vi "movimentacao_cin_inv.vi"() -> ()   [LabVIEW 2017]
doc: "The myRIO Project template acquires acceleration data from the onboard accelerometer and displays the changes of acceleration values in a waveform chart."
uses:
  <vilib>/myRIO/Instrument Drivers/Onboard IO/PWM/PWM.lvlib
  <vilib>/myRIO/Instrument Drivers/Onboard IO/PWM/typedefs/PWM Configuration.ctl
  <vilib>/myRIO/Common/Instrument Driver Framework/myRIO v1.0/PWM/typedefs/PWM Channels Enum.ctl
  <vilib>/myRIO/Common/Instrument Driver Framework/Utilities/typedefs/Generic FPGA Reference.ctl
  <vilib>/myRIO/Common/Instrument Driver Framework/Utilities/typedefs/myRIO v1.0 Reference.ctl
  <vilib>/myRIO/Common/Instrument Driver Framework/Utilities/typedefs/Hardware Version Enum.ctl
  <vilib>/myRIO/Common/Instrument Driver Framework/Utilities/typedefs/myRIO Generic Hardware Reference.ctl
  <vilib>/myRIO/Instrument Drivers/Onboard IO/PWM/typedefs/PWM Reference.ctl
  <vilib>/userdefined/High Color/nirio_resource_hc.ctl
  <vilib>/myRIO/Common/Instrument Driver Framework/myRIO v1.0/PWM/vis/myRIO v1.1 Open PWM.vi
  <vilib>/myRIO/Instrument Drivers/Onboard IO/PWM/vis/myRIO PWM Open.xnode
  <vilib>/Analysis/Matrix/Datatypes/RealMatrix.ctl
  <vilib>/Analysis/Matrix/NI_Matrix.lvlib
panel:
  in  "número de pontos que a matriz deve retornar":i64
  in  "String 2":string="(151,57;2,89;11,57);(245,79;-185,54;30);(126,28;-267,6;41,68);(43,16; -253,15;220,9);(-167,79;-132,49;100)"
  out "output array":T1
  out "appended array 2":dbl[](array[numeric])
  out "logical AND":bool
  out "x = y?":bool[](array[boolean])
  out "POS_E_ORIEN_HOME":dbl[](array[numeric])
  out "ANG_POSI_E_ORIEN_HOME":dbl[](array[numeric])
  out "CURRENT POSITIONS OF THE MOTORS":dbl[](array[numeric])
  in  "angulo_garra":dbl(knob) scale=-180.0..180.0
  out "POSITIONS SEQUENCE":T1
  in  "Duty Cycle Abert":dbl=0.04 format="%#_13g"
  out "Actuator 2":bool
  in  "Actuator":bool
  in  "Conveyor speed (mm/s)":dbl(slide)=200.0 step=1.0 scale=0.0..350.0
  out "indexador":i32
  out "Objeto detectado":bool
  out "Manipulando":bool
  out "Está em Home":bool
  out "Posicao_desejada":bool
  in  "Home":bool
  in  "error in (no error)":errorcluster
  in  "PARAR":bool
  in  "POSITION VECTOR":dbl[](array[numeric])
  # "ROTINA DE CONTROLE DO PROTÓTIPO DE FMS"
  # "COMANDO DE POSIÇÃO\nATUAL DOS MOTORES"
  # "OPERATION STATUS"
  # "ÂNGULOS DE JUNTAS"
  # "THETA 1"
  # "MOTOR 1"
  # "HOME"
  # "THETA 2"
  # "MOTOR 2"
  # "DESIRED POSITION"
  # "THETA 3"
  # "MOTOR 3"
  # "OBJECT DETECTED"
  # "THETA 4"
  # "MOTOR 4"
  # "MANIPULATING"
  # "THETA 5"
  # "MOTOR 5"
  # "ACTUATOR"
  # "MOTOR 6"
  # "VELOCIDADE DA ESTEIRA (mm/s)"
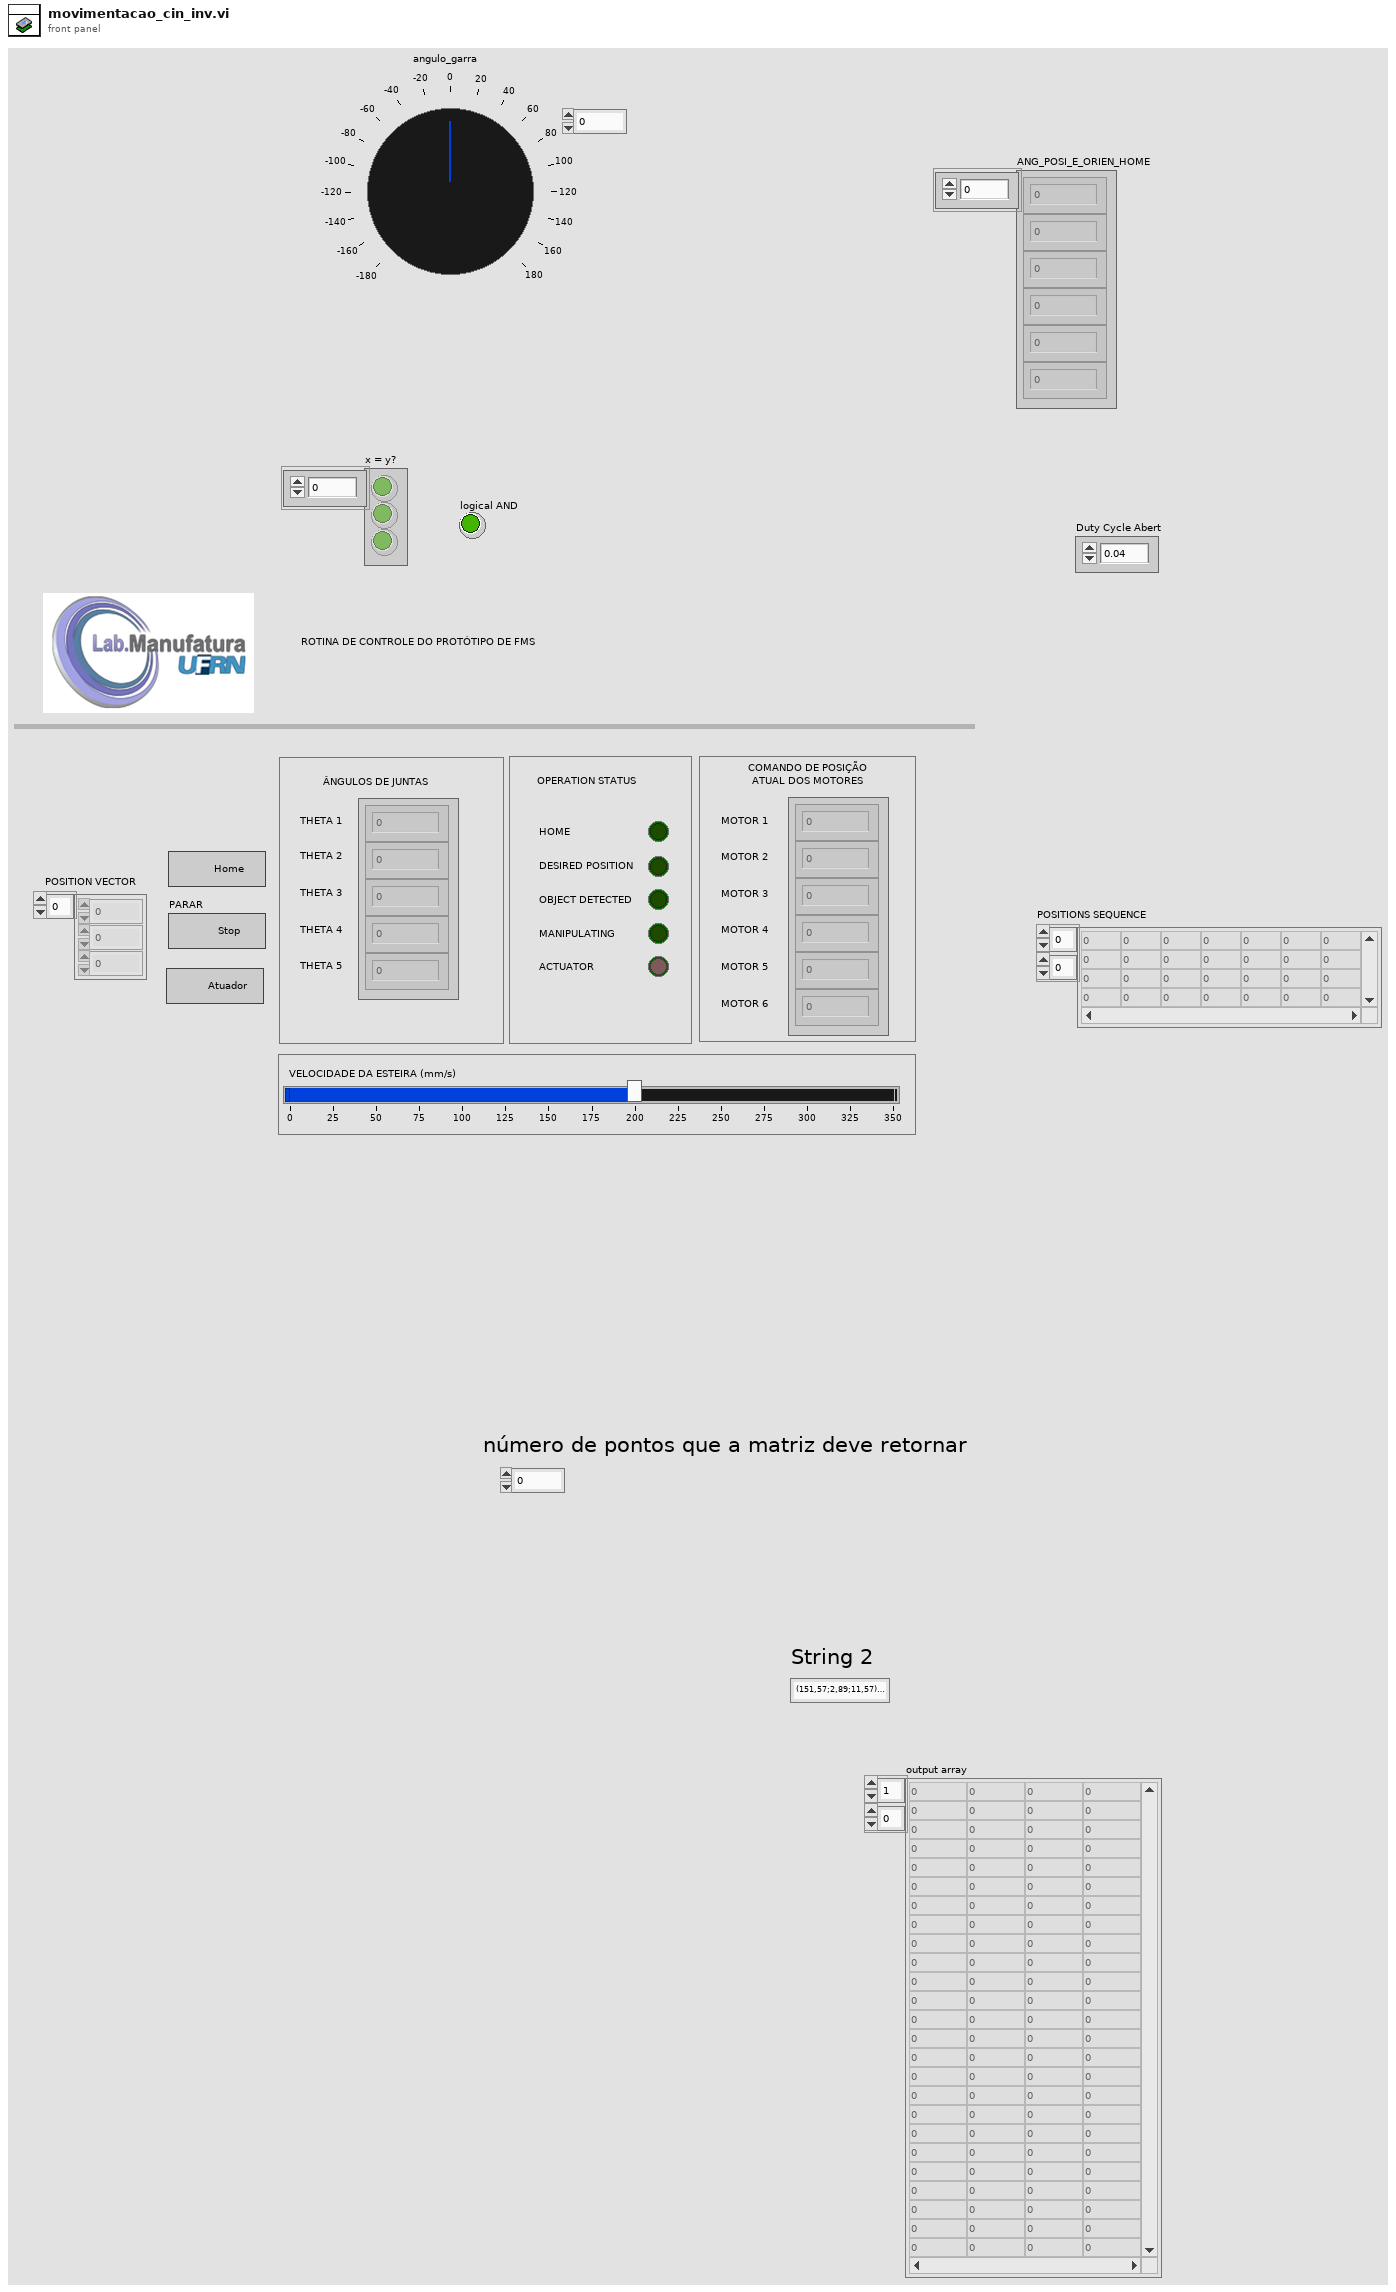
[diagram p1: front panel]
types:
  T1 = typedef "NI_Matrix.lvlib/RealMatrix.ctl" = dbl[][]
  T2 = cluster{"theta 1":dbl, "theta 2":dbl, "theta 3":dbl, "theta5":dbl, "theta4":dbl}
  T3 = typedef "nirio_resource_hc.ctl" = tag
  T4 = typedef "Hardware Version Enum.ctl" = enum16{"Unknown", "myRIO-1900", "myRIO-1950", "roboRIO", "NI ELVIS RIO CM"}
  T5 = typedef "PWM.lvlib/PWM Reference.ctl" = cluster{"myRIO Reference":T6, "PWM Channels Enum":T9, "PWM Configuration":T10}
  T6 = typedef "myRIO Generic Hardware Reference.ctl" = cluster{"myRIO Model":T4, "myRIO Hardware Reference":T7}
  T7 = typedef "myRIO v1.0 Reference.ctl" = cluster{"Generic FPGA Reference":T8, "Allow multiple opens":bool}
  T8 = typedef "Generic FPGA Reference.ctl" = refnum<k20>
  T9 = typedef "PWM Channels Enum.ctl" = enum16{"Not Connected", "C/PWM0", "C/PWM1", "A/PWM0", "A/PWM1", "A/PWM2", "B/PWM0", "B/PWM1", "B/PWM2", "PWM/PWM0", "PWM/PWM1", "PWM/PWM2", "PWM/PWM3", "PWM/PWM4", "PWM/PWM5", "PWM/PWM6", "PWM/PWM7", "PWM/PWM8", "PWM/PWM9"}
  T10 = typedef "PWM.lvlib/PWM Configuration.ctl" = cluster{"Frequency":dbl, "Duty Cycle":dbl}
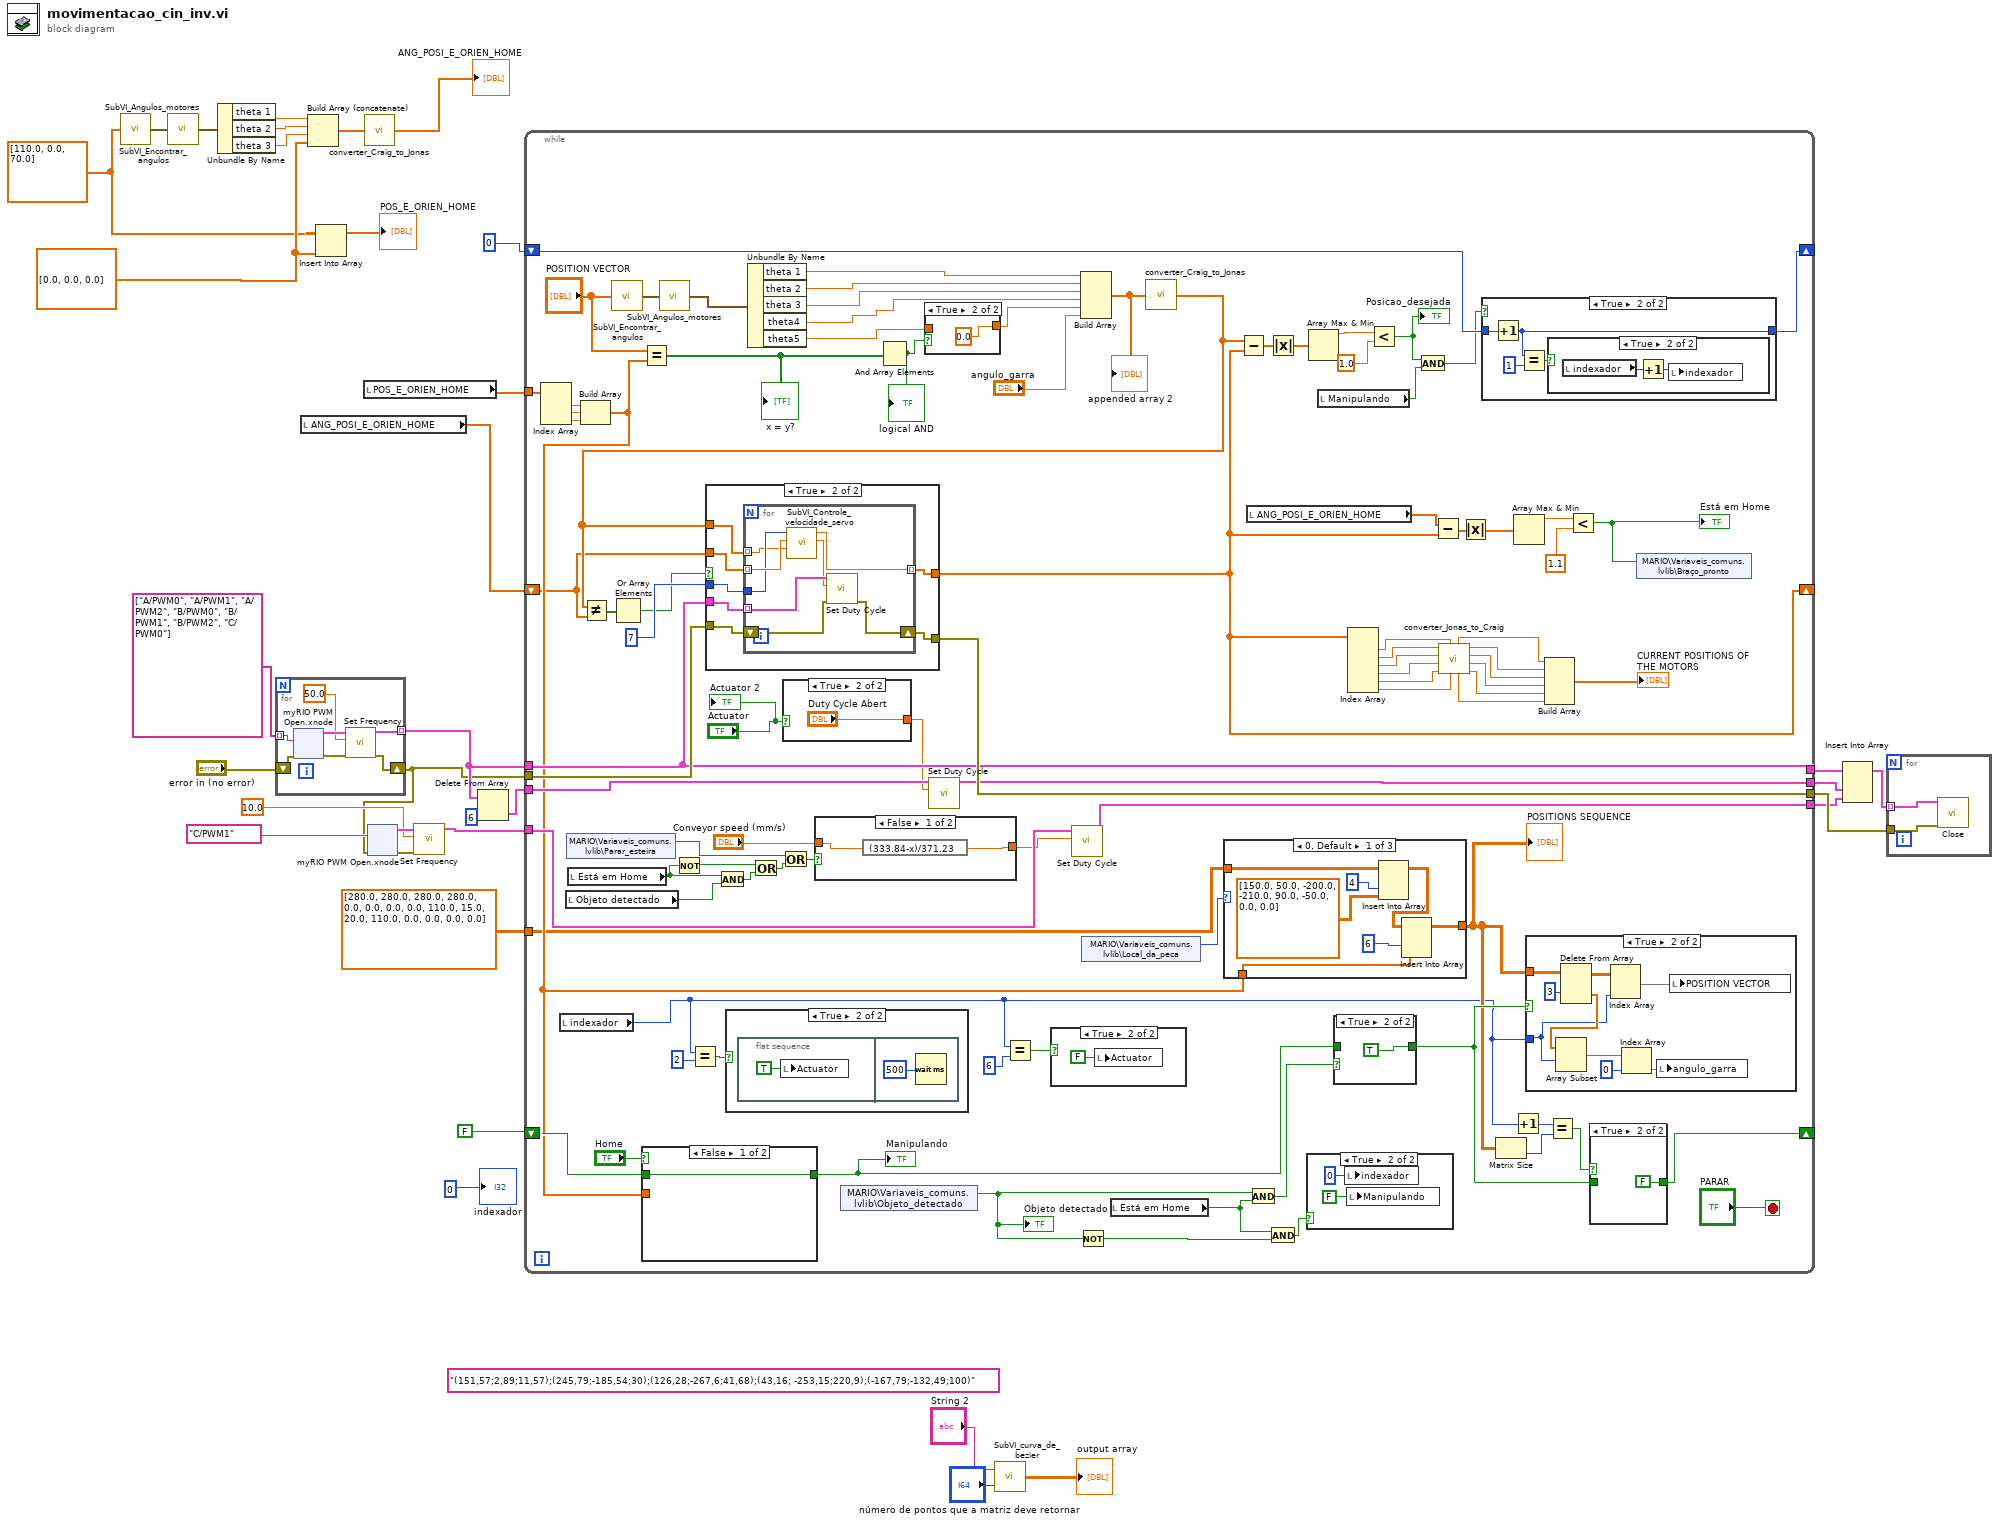
[diagram p0: block diagram]
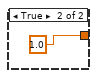
[diagram p2: hidden frame]
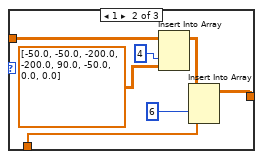
[diagram p4: hidden frame]
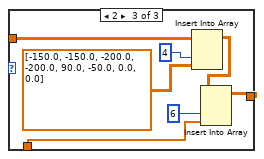
[diagram p5: hidden frame]
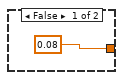
[diagram p7: hidden frame]
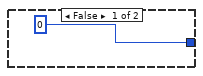
[diagram p11: hidden frame]
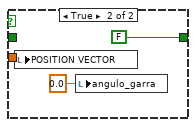
[diagram p15: hidden frame]
diagram:
  (unwired) "(151,57;2,89;11,57);(245,79;-185,54;30);(126,28;-267,6;41,68);(43,16; -253,15;220,9);(-167,79;-132,49;100)" ("String 2")
  w12 = dbl[] [0.0, 0.0, 0.0] ("vetor_P")
  w6 = dbl[] [110.0, 0.0, 70.0] ("vetor_P")
  n1 = call "SubVI_Encontrar_angulos.vi"("vetor_P"=w6) -> ("ângulos de Juntas"=w5:T2)
  n2 = call "SubVI_Angulos_motores.vi"("input cluster"=w5) -> ("output cluster"=w4:T2)
  n3 = Unbundle By Name(w4) -> ("theta 1"=w16:dbl, "theta 2"=w15:dbl, "theta 3"=w14:dbl)
  n4 = for {
    tunnel: tag[] ["A/PWM0", "A/PWM1", "A/PWM2", "B/PWM0", "B/PWM1", "B/PWM2", "C/PWM0"] -> [w39] mode=indexing
    tunnel: [w38] -> w29 mode=indexing
    shift-right: [w37] -> w18
    shift-left: "error in (no error)" -> [w36]
    n5 = xnode ("myRIO PWM Open.xnode")("error in (no error)"=w36, "Channel Name"=w39) -> ("error out"=w40:errorcluster, "PWM Ref Out"=w42:T5)  [unwired: 1 in]
    n6 = call <vilib>:"Set Frequency.vi"("error in (no error)"=w40, "Frequency [Hz]"=50.0, "PWM Ref In"=w42) -> ("error out"=w37:errorcluster, "PWM Ref Out"=w38:T5)  [unwired: 6 in]
  }
  n7 = local read "ANG_POSI_E_ORIEN_HOME"() -> (w13:dbl[])
  n8 = Build Array (concatenate)(w16, w15, w14, w12) -> (w8:dbl[])
  n9 = Insert Into Array(array=w6, new element=w12) -> (→"POS_E_ORIEN_HOME":dbl[])  [unwired: 1 in]
  n10 = local read "POS_E_ORIEN_HOME"() -> (w10:dbl[])
  n11 = call "converter_Craig_to_Jonas.vi"("array"=w8) -> ("appended array"=→"ANG_POSI_E_ORIEN_HOME":dbl[])
  n12 = xnode "myRIO PWM Open.xnode"("error in (no error)"=w18, "Channel Name"=tag "C/PWM1") -> ("error out"=w22:errorcluster, "PWM Ref Out"=w23:T5)  [unwired: 1 in]
  n13 = call <vilib>:"Set Frequency.vi"("error in (no error)"=w22, "Frequency [Hz]"=10.0, "PWM Ref In"=w23) -> ("PWM Ref Out"=w19:T5)  [unwired: 6 in, 1 out]
  n14 = Delete From Array(array=w29, index=6) -> (deleted portion=w27:T5)  [unwired: 1 in, 1 out]
  n15 = while {
    tunnel: [w149] -> w35
    shift-right: [w67] -> _
    shift-left: w13 -> [w59]
    tunnel: w18 -> [w147]
    tunnel: w29 -> [w146]
    tunnel: [w146] -> w26
    shift-right: [w128] -> _
    shift-left: FALSE -> [w129]
    shift-right: [w138] -> _
    shift-left: u32 0 ("ms to wait (braço)") -> [w137]
    tunnel: w27 -> [w122]
    tunnel: [w121] -> w25
    tunnel: w19 -> [w117]
    tunnel: [w113] -> w17
    tunnel: w10 -> [w81]
    tunnel: T1 [[280.0, 280.0, 280.0, 280.0], [0.0, 0.0, 0.0, 0.0], [110.0, 15.0, 20.0, 110.0], [0.0, 0.0, 0.0, 0.0]] ("matrix 2") -> [w77]
    stop <- "PARAR" stop-if-true
    n16 = Index Array(array=w81) -> (element #1=w84:dbl, element #2=w83:dbl, element #3=w82:dbl)  [unwired: 3 in]
    n17 = local read "indexador"() -> (w69:i32)
    n18 = local read "Objeto detectado"() -> (w110:bool)
    n19 = shared-variable "MARIO\\Variaveis_comuns.lvlib\\Parar_esteira"() -> (w112:bool)  [unwired: 1 in, 1 out]
    n20 = local read "Está em Home"() -> (w107:bool)
    n21 = Build Array(w84, w83, w82) -> (w80:dbl[])
    n22 = call "SubVI_Encontrar_angulos.vi"("vetor_P"="POSITION VECTOR") -> ("ângulos de Juntas"=w64:T2)
    n23 = Equal?(x="POSITION VECTOR", y=w80) -> (x = y?=w125:bool[])
    "x = y?" <- w125
    n24 = case shown="False" "Home" {
      tunnel: w80 -> [_ w207]
      tunnel: w129 -> [w204 _]
      tunnel: [w204 FALSE ("Manipulando")] -> w66
      frame False {
      }
      frame True {
        n25 = local write "POSITION VECTOR"(w207) -> ()
        n26 = local write "angulo_garra"(0.0 ("angulo_garra")) -> ()
      }
    }
    "Manipulando" <- w66
    n27 = call "SubVI_Angulos_motores.vi"("input cluster"=w64) -> ("output cluster"=w63:T2)
    n28 = Not(x=w107) -> (.not. x?=w108:bool)
    n29 = Equal?(x=w69, y=2 ("x")) -> (x = y?=w119:bool)
    n30 = And(x=w107, y=w110) -> (x .and. y?=w109:bool)
    n31 = case shown="True" w119 {
      frame False {
      }
      frame True {
        n32 = flat-sequence {
          frame #0 {
            n33 = local write "Actuator"(TRUE ("Actuator")) -> ()
          }
          frame #1 {
            n34 = Wait (ms)(milliseconds to wait=u32 500) -> ()  [unwired: 1 out]
          }
        }
      }
    }
    n35 = Unbundle By Name(w63) -> ("theta 1"=w90:dbl, "theta 2"=w89:dbl, "theta 3"=w88:dbl, "theta4"=w62:dbl, "theta5"=w61:dbl)
    n36 = Or(x=w108, y=w109) -> (x .or. y?=w106:bool)
    n37 = Or(x=w112, y=w106) -> (x .or. y?=w114:bool)
    n38 = case shown="True" "Actuator" {
      tunnel: [0.08 ("Duty Cycle Abert") "Duty Cycle Abert"] -> w120
      frame False {
      }
      frame True {
      }
    }
    n39 = case shown="False" w114 {
      tunnel: [w152 1.0 ("Duty Cycle")] -> w116
      tunnel: "Conveyor speed (mm/s)" -> [w151 _]
      frame False {
        n40 = expression code="(333.84-x)/371.23"(w151) -> (w152:dbl)
      }
      frame True {
      }
    }
    n41 = shared-variable "MARIO\\Variaveis_comuns.lvlib\\Objeto_detectado"() -> (w104:bool)  [unwired: 1 in, 1 out]
    "Objeto detectado" <- w104
    n42 = And Array Elements(Boolean array=w125) -> (logical AND=w124:bool)
    "logical AND" <- w124
    n43 = case shown="True" w124 {
      tunnel: [w180 0.0 ("theta5")] -> w87
      tunnel: w61 -> [w180 _]
      frame False {
      }
      frame True {
      }
    }
    n44 = call <vilib>:"Set Duty Cycle.vi"("Duty Cycle"=w120, "PWM Ref In"=w122) -> ("PWM Ref Out"=w121:T5)  [unwired: 7 in, 1 out]
    n45 = Equal?(x=w69, y=6 ("x")) -> (x = y?=w118:bool)
    n46 = case shown="True" w118 {
      frame False {
      }
      frame True {
        n47 = local write "Actuator"(FALSE ("Actuator")) -> ()
      }
    }
    n48 = call <vilib>:"Set Duty Cycle.vi"("Duty Cycle"=w116, "PWM Ref In"=w117) -> ("PWM Ref Out"=w113:T5)  [unwired: 7 in, 1 out]
    n49 = Not(x=w104) -> (.not. x?=w75:bool)
    n50 = Build Array(w90, w89, w88, w62, w87, "angulo_garra") -> (w86:dbl[])
    "appended array 2" <- w86
    n51 = shared-variable "MARIO\\Variaveis_comuns.lvlib\\Local_da_peca"() -> (w105:i8)  [unwired: 1 in, 1 out]
    n52 = local read "Está em Home"() -> (w76:bool)
    n53 = call "converter_Craig_to_Jonas.vi"("array"=w86) -> ("appended array"=w79:dbl[])
    n54 = Not Equal?(x=w79, y=w59) -> (x != y?=w145:bool[])
    n55 = Or Array Elements(Boolean array=w145) -> (logical OR=w144:bool)
    n56 = case shown="True" w144 {
      tunnel: [w208 w216] -> w149
      tunnel: w147 -> [w208 w215]
      tunnel: w146 -> [_ w214]
      tunnel: w59 -> [w209 w213]
      tunnel: [w209 w211] -> w67
      tunnel: u32 7 ("ms to wait (braço)") -> [_ w212]
      tunnel: w79 -> [_ w210]
      frame False {
      }
      frame True {
        n57 = for {
          tunnel: w214 -> [w222] mode=indexing
          tunnel: w213 -> [w221] mode=indexing
          tunnel: w212 -> [w219]
          tunnel: [w218] -> w211 mode=indexing
          tunnel: w210 -> [w217] mode=indexing
          shift-right: [w224] -> w216
          shift-left: w215 -> [w223]
          n58 = call "SubVI_Controle_velocidade_servo.vi"("Posição Desejada"=w217, "Posição"=w221, "milliseconds to wait"=w219) -> ("Duty Cycle"=w220:dbl, "Posição"=w218:dbl)  [unwired: 7 in]
          n59 = call <vilib>:"Set Duty Cycle.vi"("error in (no error)"=w223, "Duty Cycle"=w220, "PWM Ref In"=w222) -> ("error out"=w224:errorcluster)  [unwired: 6 in, 1 out]
        }
      }
    }
    n60 = case shown="0, Default" w105 {
      tunnel: w77 -> [w155 w164 w172]
      tunnel: w80 -> [w157 w162 w171]
      tunnel: [w156 w163 w170] -> w74
      frame 0, Default {
        n61 = Insert Into Array(array=w155, index (col)=4 ("disabled index (col)"), new element=T1 [[150.0, 50.0], [-200.0, -210.0], [90.0, -50.0], [0.0, 0.0]] ("matrix")) -> (w159:T1)  [unwired: 1 in]
        n62 = Insert Into Array(array=w159, index (col)=6 ("disabled index (col)"), new element=w157) -> (w156:T1)  [unwired: 1 in]
      }
      frame 1 {
        n63 = Insert Into Array(array=w164, index (col)=4 ("disabled index (col)"), new element=T1 [[-50.0, -50.0], [-200.0, -200.0], [90.0, -50.0], [0.0, 0.0]] ("matrix 2")) -> (w166:T1)  [unwired: 1 in]
        n64 = Insert Into Array(array=w166, index (col)=6 ("disabled index (col)"), new element=w162) -> (w163:T1)  [unwired: 1 in]
      }
      frame 2 {
        n65 = Insert Into Array(array=w172, index (col)=4 ("disabled index (col)"), new element=T1 [[-150.0, -150.0], [-200.0, -200.0], [90.0, -50.0], [0.0, 0.0]] ("matrix 3")) -> (w169:T1)  [unwired: 1 in]
        n66 = Insert Into Array(array=w169, index (col)=6 ("disabled index (col)"), new element=w171) -> (w170:T1)  [unwired: 1 in]
      }
    }
    "POSITIONS SEQUENCE" <- w74
    n67 = Subtract(x=w79, y=w67) -> (x-y=w143:dbl[])
    n68 = local read "ANG_POSI_E_ORIEN_HOME"() -> (w85:dbl[])
    n69 = And(x=w104, y=w76) -> (x .and. y?=w140:bool)
    n70 = Absolute Value(x=w143) -> (abs(x)=w142:dbl[])
    n71 = And(x=w76, y=w75) -> (x .and. y?=w134:bool)
    n72 = case shown="True" w134 {
      frame False {
      }
      frame True {
        n73 = local write "indexador"(0 ("indexador")) -> ()
        n74 = local write "Manipulando"(FALSE ("Manipulando")) -> ()
      }
    }
    n75 = Array Max & Min(array=w142) -> (max value=w78:dbl)  [unwired: 3 out]
    n76 = local read "Manipulando"() -> (w136:bool)
    n77 = case shown="True" w140 {
      tunnel: [w202 TRUE] -> w127
      tunnel: w66 -> [w202 _]
      frame False {
      }
      frame True {
      }
    }
    n78 = Index Array(array=w67) -> (element #1=w103:dbl, element #2=w102:dbl, element #3=w101:dbl, element #4=w100:dbl, element #5=w99:dbl, element #6=w98:dbl)  [unwired: 6 in]
    n79 = Less?(x=w78, y=1.0) -> (x < y?=w68:bool)
    "Posicao_desejada" <- w68
    n80 = And(x=w68, y=w136) -> (x .and. y?=w135:bool)
    n81 = Subtract(x=w85, y=w67) -> (x-y=w133:dbl[])
    n82 = call "converter_Jonas_to_Craig.vi"("theta6Jonas"=w98, "theta1Jonas"=w103, "theta5Jonas"=w99, "theta4Jonas"=w100, "theta3Jonas"=w101, "theta2Jonas"=w102) -> ("theta5Craig"=w93:dbl, "theta4Craig"=w94:dbl, "theta3Craig"=w95:dbl, "theta2Craig"=w96:dbl, "theta6Craig"=w92:dbl, "theta1Craig"=w97:dbl)
    n83 = Absolute Value(x=w133) -> (abs(x)=w132:dbl[])
    n84 = case shown="True" w135 {
      tunnel: w137 -> [_ w197]
      tunnel: [u32 0 ("ms to wait (braço)") w196] -> w138
      frame False {
      }
      frame True {
        n85 = Increment(x=w197) -> (x+1=w196:u32)
        n86 = Equal?(x=w196, y=u32 1) -> (x = y?=w194:bool)
        n87 = case shown="True" w194 {
          frame False {
          }
          frame True {
            n88 = local read "indexador"() -> (w199:i32)
            n89 = Increment(x=w199) -> (x+1=w198:i32)
            n90 = local write "indexador"(w198) -> ()
          }
        }
      }
    }
    n91 = Matrix Size(0:w74) -> (2:w72:i32)  [unwired: 1 out]
    n92 = Increment(x=w69) -> (x+1=w73:i32)
    n93 = Array Max & Min(array=w132) -> (max value=w131:dbl)  [unwired: 3 out]
    n94 = case shown="True" w127 {
      tunnel: w74 -> [_ w191]
      tunnel: w69 -> [_ w184]
      frame False {
      }
      frame True {
        n95 = Delete From Array(array=w191, index (row)=3) -> (deleted portion=w185:dbl[], array with subset deleted=w189:T1)  [unwired: 2 in]
        n96 = Array Subset(array=w185, index=w184) -> (w188:dbl[])  [unwired: 1 in]
        n97 = Index Array(array=w189, index (col)=w184) -> (element=w192:dbl[])  [unwired: 1 in]
        n98 = Index Array(array=w188, index=0) -> (element=w186:dbl)
        n99 = local write "angulo_garra"(w186) -> ()
        n100 = local write "POSITION VECTOR"(w192) -> ()
      }
    }
    n101 = Build Array(w97, w96, w95, w94, w93, w92) -> (→"CURRENT POSITIONS OF THE MOTORS":dbl[])
    n102 = Equal?(x=w73, y=w72) -> (x = y?=w126:bool)
    n103 = Less?(x=w131, y=1.1) -> (x < y?=w111:bool)
    "Está em Home" <- w111
    n104 = case shown="True" w126 {
      tunnel: [w182 FALSE ("Manipulando")] -> w128
      tunnel: w127 -> [w182 _]
      frame False {
      }
      frame True {
      }
    }
    n105 = shared-variable "MARIO\\Variaveis_comuns.lvlib\\Braço_pronto"(w111) -> ()  [unwired: 1 in, 1 out]
    "Actuator 2" <- "Actuator"
  }
  n106 = call "SubVI_curva_de_bezier.vi"("número de pontos que a matriz deve retornar"="número de pontos que a matriz deve retornar", "String in"="String 2") -> ("matrix"=→"output array":T1)
  n107 = Insert Into Array(array=w26, new element #1=w25, new element #2=w17) -> (w24:T5[])  [unwired: 1 in]
  n108 = for {
    tunnel: w35 -> [w226]
    tunnel: w24 -> [w225] mode=indexing
    n109 = call <vilib>:"Close.vi"("error in (no error)"=w226, "PWM Ref In"=w225) -> ()  [unwired: 9 in, 1 out]
  }
  "indexador" <- 0
